vi "Generate_no.vi"(8 "error in (no error)":errorcluster, 11 "Button_transfer in":refnum<class "Button_transfer.lvclass">) -> (0 "error out":errorcluster, 3 "Button_transfer out":refnum<class "Button_transfer.lvclass">)   [LabVIEW 2025, in "Button_transfer.lvlib" / "Button_transfer.lvclass"]
uses:
  Button_transfer.lvclass
  Button_transfer.lvclass/Button_transfer.ctl
  <vilib>/numeric/Random Number (Range) U64.vi
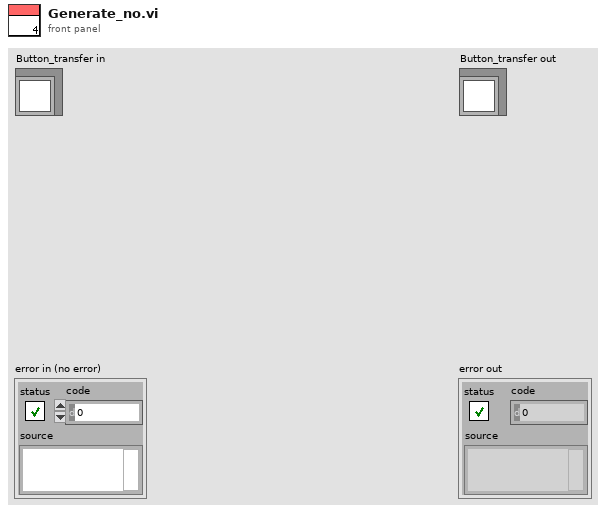
[diagram p1: front panel]
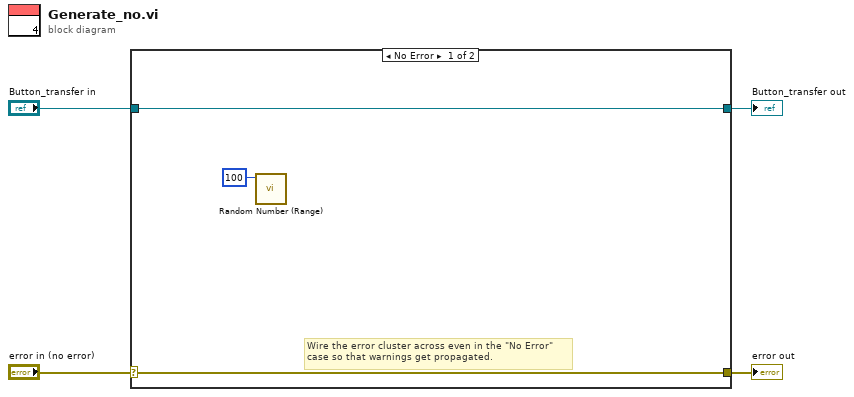
[diagram p0: block diagram]
diagram:
  n1 = case shown="No Error" "error in (no error)" {
    selector: "error in (no error)" -> [w6 w9]
    tunnel: [w6 w9] -> w3
    tunnel: [w7 w8] -> w1
    tunnel: "Button_transfer in" -> [w7 w8]
    frame No Error {
      # "Wire the error cluster across even in the \"No Error\"\ncase so that warnings get propagated."
      n2 = call-poly <vilib>:"Random Number (Range).vi"("upper bound (100)"=u64 100) -> ()  [unwired: 10 in, 1 out]
    }
    frame Error {
    }
  }
  "error out" <- w3
  "Button_transfer out" <- w1
